vi "_MDPtr Push Ptr Back to CacheQueue.vi"(8 "error in":errorcluster, 10 "Cache Length":i32, 11 "MDPtr":T1) -> (0 "error out":errorcluster)   [LabVIEW 2017, in "MDPtr.lvlib"]
uses:
  MDPtr.lvlib
  MDPtr TypeDef/MDPtr.ctl
  _MDPtrMgr/MDPtrMgr.lvclass
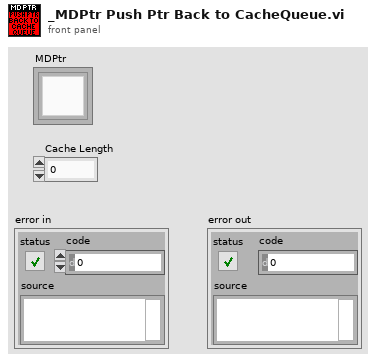
[diagram p1: front panel]
types:
  T1 = typedef "MDPtr.lvlib/MDPtr.ctl" = refnum<k1>
  T2 = typedef "MDPtr.lvlib/MDPtr Queue.ctl" = refnum<queue>
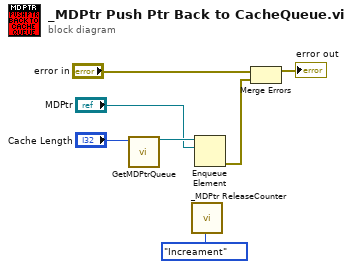
[diagram p0: block diagram]
diagram:
  n1 = call "GetMDPtrQueue.vi"("MemoryLength"="Cache Length") -> ("MDPtrQueue"=w6:T2)  [unwired: 8 in, 2 out]
  n2 = call "_MDPtr ReleaseCounter.vi"("Oper(Get)"=enum16{"GET", "Increament", "decreament"}."Increament") -> ()  [unwired: 9 in, 2 out]
  n3 = Enqueue Element(queue=w6, element="MDPtr") -> (error out=w3:errorcluster)  [unwired: 2 in, 2 out]
  n4 = Merge Errors("error in", w3) -> (→"error out":errorcluster)
